vi "TestExec.Merge Variables from VarientAttr and 2D Str.vi"(10 "Vars In 2D":string[][](array[string]), 11 "Vars In":variant) -> (2 "Vars Out 2D":string[][](array[string]), 3 "Vars Out":variant)   [LabVIEW 2018]
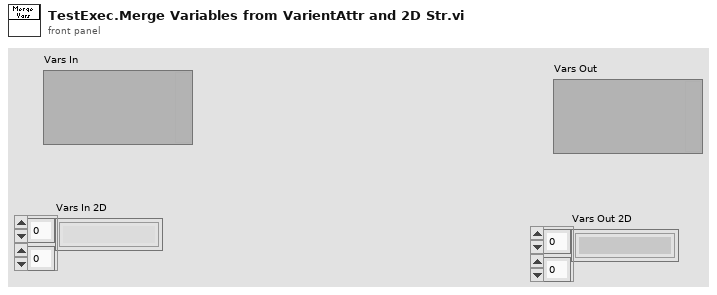
[diagram p1: front panel]
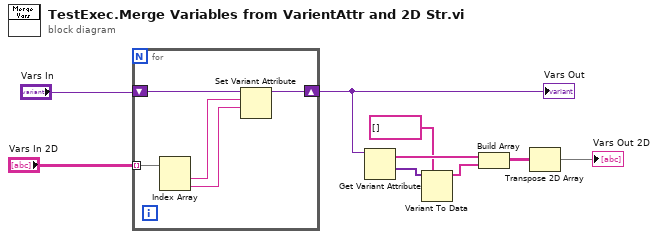
[diagram p0: block diagram]
diagram:
  n1 = for {
    tunnel: "Vars In 2D" -> [w14] mode=indexing
    shift-right: [w10] -> w2
    shift-left: "Vars In" -> [w13]
    n2 = Index Array(array=w14) -> (element #1=w12:string, element #2=w11:string)  [unwired: 2 in]
    n3 = Set Variant Attribute(Variant=w13, name=w12, value=w11) -> (Variant out=w10:variant)  [unwired: 1 in, 2 out]
  }
  "Vars Out" <- w2
  n4 = Get Variant Attribute(Variant=w2) -> (names=w7:string[], values=w6:variant[])  [unwired: 3 in, 2 out]
  n5 = Variant To Data(type=string[] [], Variant=w6) -> (data=w4:string[])  [unwired: 1 in, 1 out]
  n6 = Build Array(w7, w4) -> (w3:string[][])
  n7 = Transpose 2D Array(2D array=w3) -> (transposed array=→"Vars Out 2D":string[][])
